vi "ExampleControl.vi"() -> ()   [LabVIEW 2017, in "Spectral Products CM110.lvlib"]
uses:
  Spectral Products CM110.lvlib
  Public/Controls/CaseSelector.ctl
panel:
  in  "Direction":bool caption="Clockwise"
  out "Rotation Speed":u16
  in  "Desired Rotation Speed":u16=1 min=1 step=1
  in  "Zero":bool
  in  "Desired Step Size":u8=1
  in  "Step":bool
  out "Step size":u8
  out "Changing grating":bool
  in  "Switch grating":bool
  out "Number of gratings":u8
  out "Groove Density":u16
  out "Blaze Wavelength":u16
  out "Current grating #":u8
  in  "Units":u8(ring)=1 items=["nm"=1, "A"=2]
  in  "Move Absolute":bool
  in  "Wavelength":u16
  out "Command not accepted":bool
  out "Error Out":errorcluster
  in  "QUIT":bool
  out "Position":cluster{"Numeric":dbl, "Units":string}
  out "Initialized":bool
  in  "VISA resource name":refnum<visa-resource-name>="COM7"
  # "CCW"
  # "CW"
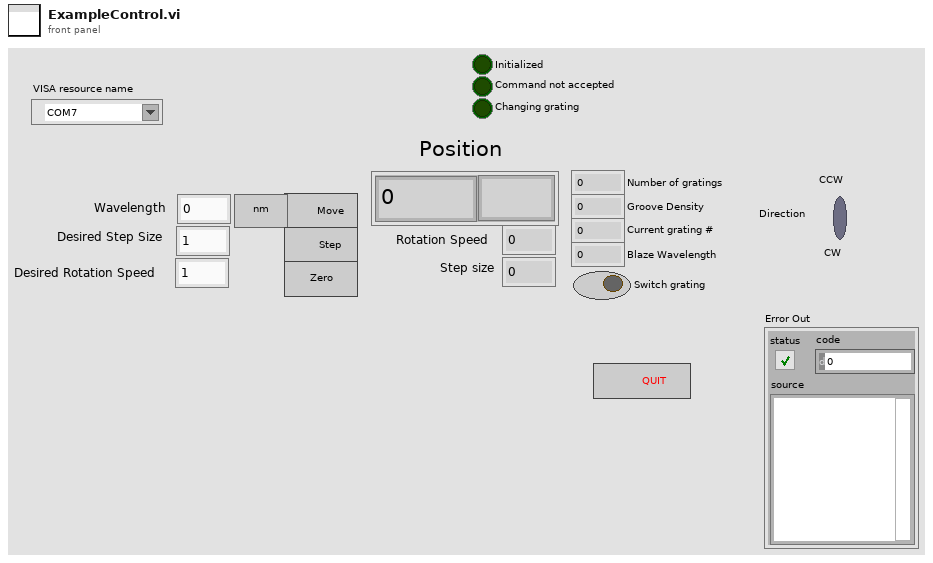
[diagram p1: front panel]
types:
  T1 = typedef "Spectral Products CM110.lvlib/CaseSelector.ctl" = enum16{"Initialize", "Get Status", "Idle", "Close", "GoTo", "Change Units", "Read Grating Info", "Change Grating", "Change Step Size", "Move One Step", "Reset", "Change Rotation Speed", "Change Rotation Direction"}
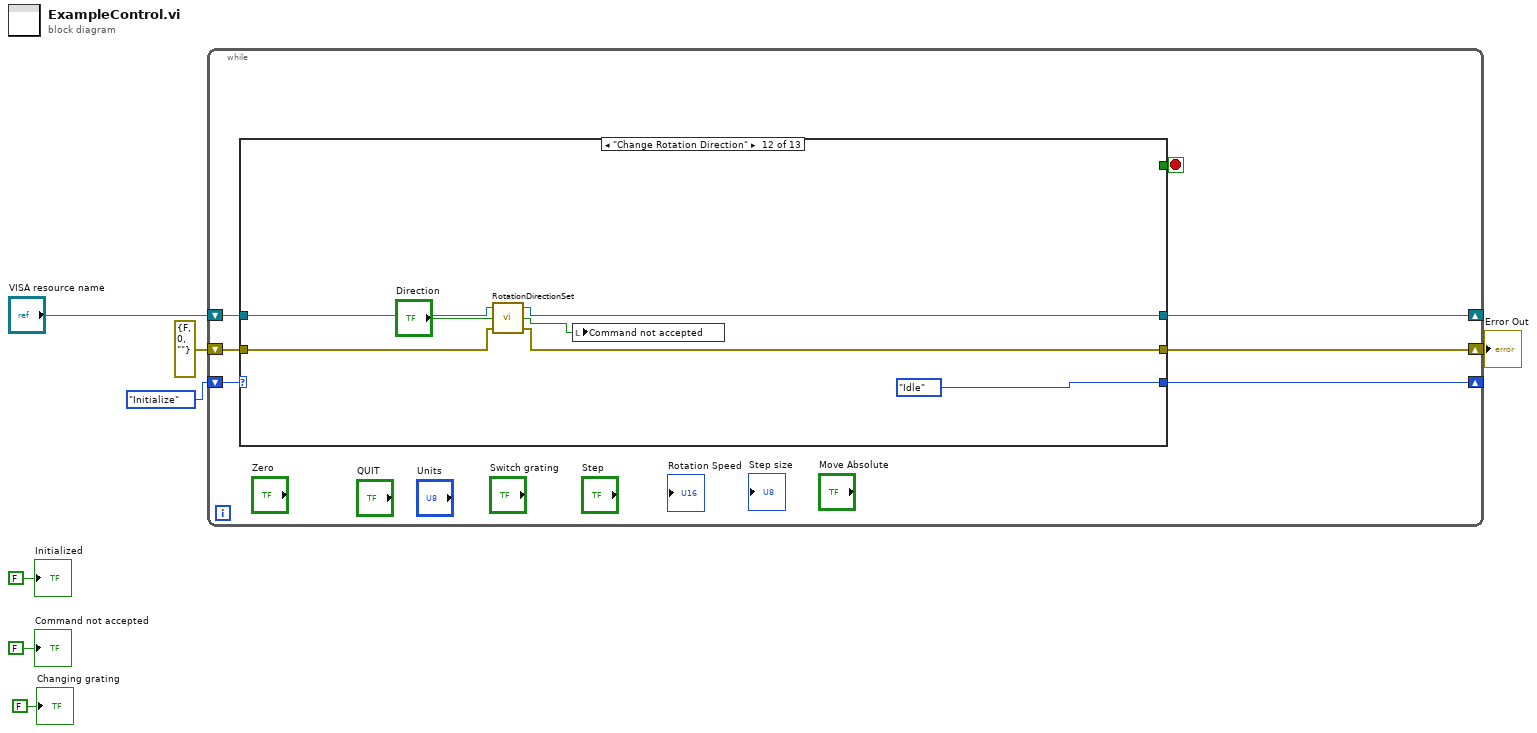
[diagram p0: block diagram]
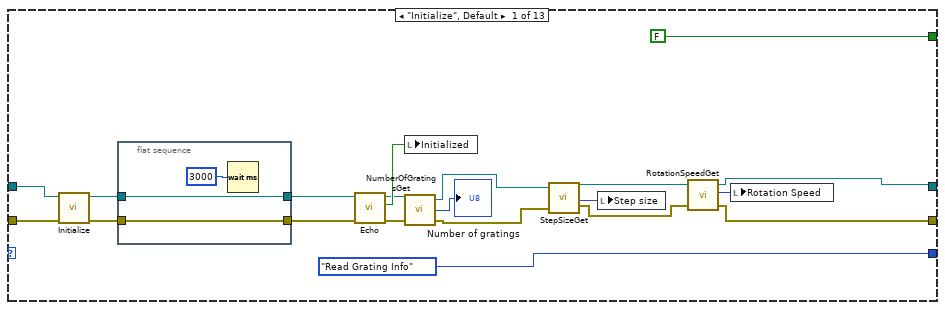
[diagram p2: hidden frame]
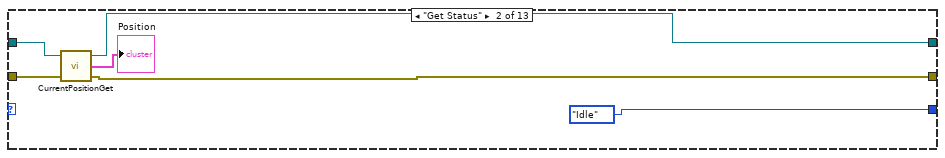
[diagram p3: hidden frame]
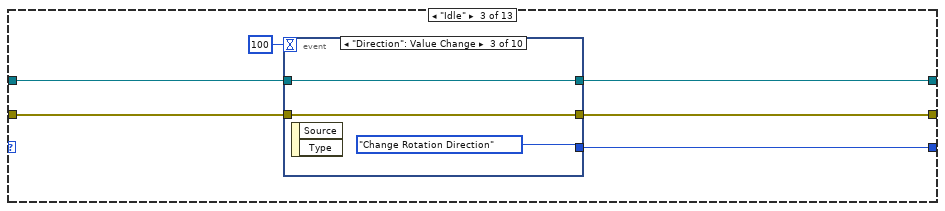
[diagram p4: hidden frame]
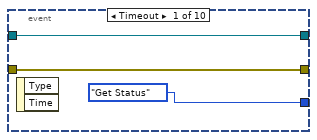
[diagram p5: hidden frame]
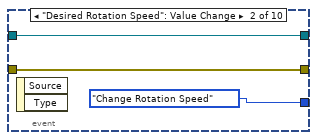
[diagram p6: hidden frame]
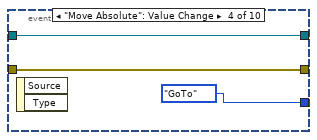
[diagram p7: hidden frame]
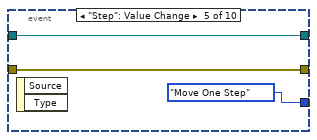
[diagram p8: hidden frame]
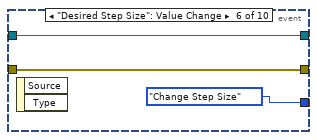
[diagram p9: hidden frame]
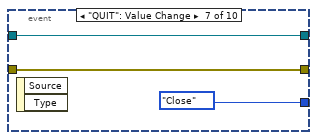
[diagram p10: hidden frame]
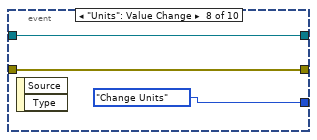
[diagram p11: hidden frame]
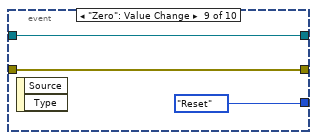
[diagram p12: hidden frame]
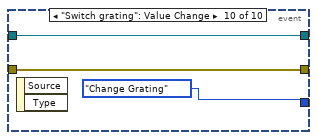
[diagram p13: hidden frame]
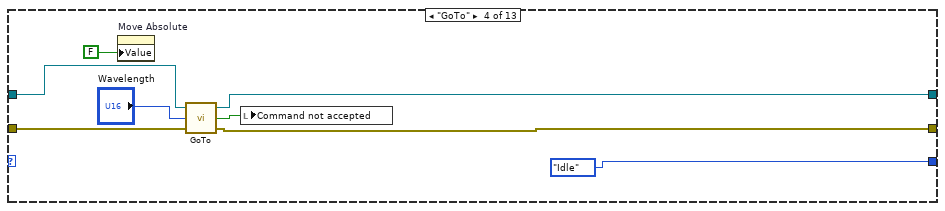
[diagram p14: hidden frame]
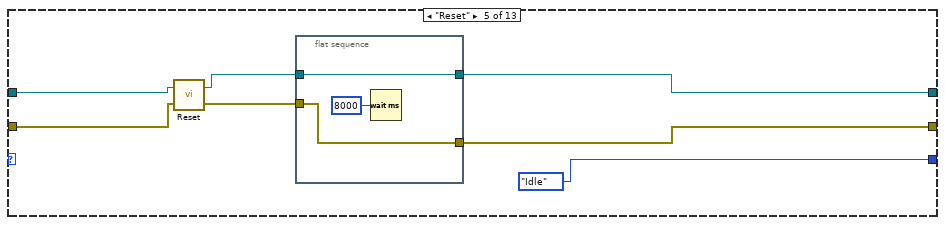
[diagram p15: hidden frame]
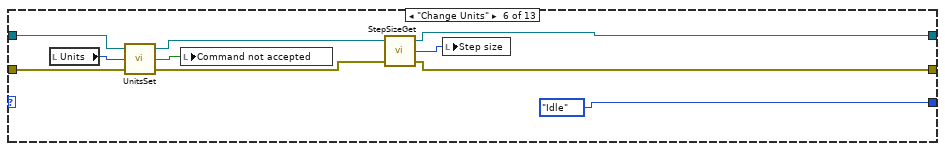
[diagram p16: hidden frame]
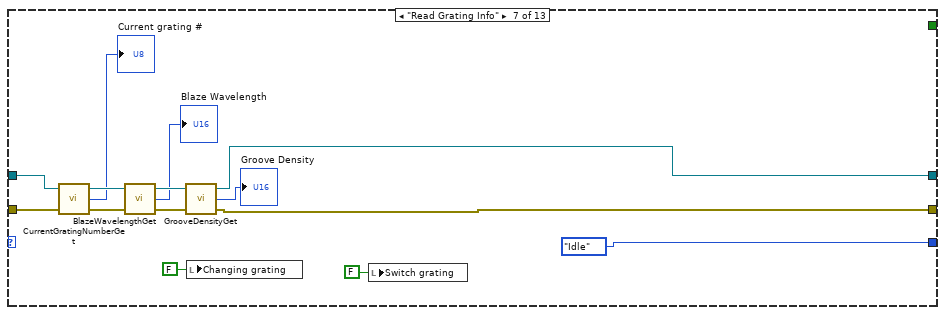
[diagram p17: hidden frame]
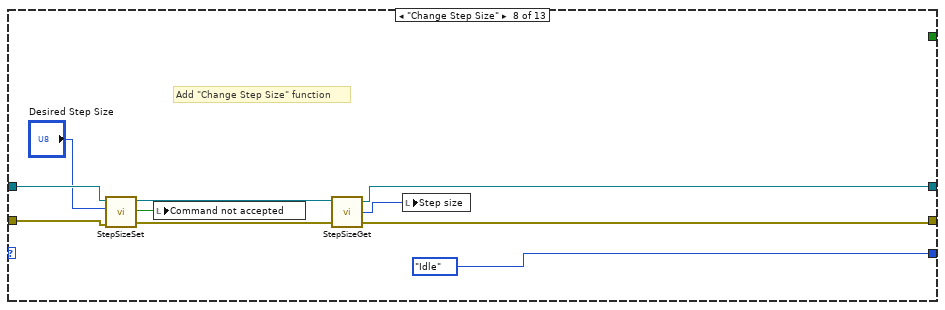
[diagram p18: hidden frame]
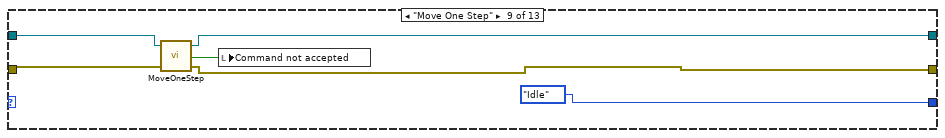
[diagram p19: hidden frame]
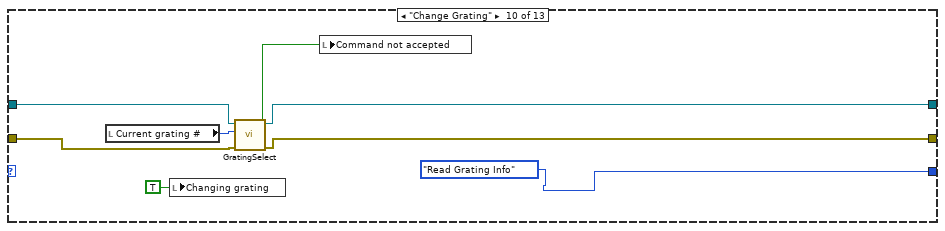
[diagram p20: hidden frame]
diagram:
  n1 = while {
    shift-right: [w11] -> _
    shift-left: "VISA resource name" -> [w14]
    shift-right: [w10] -> w3
    shift-left: errorcluster {"status"=FALSE, "code"=0, "source"=""} ("error in (no error)") -> [w13]
    shift-right: [w8] -> _
    shift-left: CaseSelector."Initialize" -> [w12]
    stop <- w9 stop-if-true
    n2 = case shown="\"Change Rotation Direction\"" w12 {
      tunnel: w14 -> [w34 w43 w46 w87 w94 w106 w121 w127 w136 w144 w155 w161 w166]
      tunnel: w13 -> [w33 w42 w44 w86 w93 w105 w120 w126 w135 w143 w153 w160 w168]
      tunnel: [w16 w40 w47 w82 w92 w99 w112 w131 w133 w141 w148 w158 w166] -> w11
      tunnel: [w15 w39 w45 w81 w90 w98 w111 w130 w132 w140 w147 w157 w165] -> w10
      tunnel: [FALSE ("Initialized") _ _ _ _ _ _ _ _ _ _ _ TRUE ("Initialized")] -> w9
      tunnel: [CaseSelector."Read Grating Info" CaseSelector."Idle" w48 CaseSelector."Idle" CaseSelector."Idle" CaseSelector."Idle" CaseSelector."Idle" CaseSelector."Idle" CaseSelector."Idle" CaseSelector."Read Grating Info" CaseSelector."Idle" CaseSelector."Idle" CaseSelector."Idle"] -> w8
      frame "Initialize", Default {
        n3 = call "Initialize.vi"("error in (no error)"=w33, "VISA resource name"=w34) -> ("error out"=w27:errorcluster, "VISA resource name out"=w28:refnum<visa-resource-name>)  [unwired: 8 in]
        n4 = flat-sequence {
          tunnel: w28 -> [w37]
          tunnel: [w37] -> w30
          tunnel: w27 -> [w36]
          tunnel: [w36] -> w29
          frame #0 {
            n5 = Wait (ms)(milliseconds to wait=u32 3000) -> ()  [unwired: 1 out]
          }
        }
        n6 = call "Echo.vi"("error in (no error)"=w29, "VISA resource name"=w30) -> ("error out"=w25:errorcluster, "ECHO"=w32:bool, "VISA resource name out"=w26:refnum<visa-resource-name>)  [unwired: 7 in]
        n7 = local write "Initialized"(w32) -> ()
        n8 = call "NumberOfGratingsGet.vi"("error in (no error)"=w25, "VISA resource name"=w26) -> ("error out"=w22:errorcluster, "Number of gratings"=→"Number of gratings":u8, "VISA resource name out"=w23:refnum<visa-resource-name>)  [unwired: 1 in]
        n9 = call "StepSizeGet.vi"("error in (no error)"=w22, "VISA resource name"=w23) -> ("error out"=w18:errorcluster, "Step size"=w20:u8, "VISA resource name out"=w19:refnum<visa-resource-name>)  [unwired: 1 in]
        n10 = local write "Step size"(w20) -> ()
        n11 = call "RotationSpeedGet.vi"("error in (no error)"=w18, "VISA resource name"=w19) -> ("error out"=w15:errorcluster, "Rotation Speed"=w17:u16, "VISA resource name out"=w16:refnum<visa-resource-name>)  [unwired: 1 in]
        n12 = local write "Rotation Speed"(w17) -> ()
      }
      frame "Get Status" {
        n13 = call "CurrentPositionGet.vi"("error in (no error)"=w42, "VISA resource name"=w43) -> ("error out"=w39:errorcluster, "Position"=→"Position":cluster{"Numeric":dbl, "Units":string}, "VISA resource name out"=w40:refnum<visa-resource-name>)  [unwired: 1 in]
      }
      frame "Idle" {
        n14 = event shown="[2] \"Direction\": Value Change" {
          selector: _ -> [_ _ _ _ _ _ _ _ _ _]
          dyn-events: _ -> [_ _ _ _ _ _ _ _ _ _]
          timeout: 100 -> [_ _ _ _ _ _ _ _ _ _]
          tunnel: [CaseSelector."Get Status" CaseSelector."Change Rotation Speed" CaseSelector."Change Rotation Direction" CaseSelector."GoTo" CaseSelector."Move One Step" CaseSelector."Change Step Size" CaseSelector."Close" CaseSelector."Change Units" CaseSelector."Reset" CaseSelector."Change Grating"] -> w48
          tunnel: [w52 w55 w56 w61 w62 w66 w70 w73 w76 w79] -> w47
          tunnel: w46 -> [w52 w55 w56 w61 w62 w66 w70 w73 w76 w79]
          tunnel: [w51 w54 w57 w60 w63 w65 w69 w72 w75 w78] -> w45
          tunnel: w44 -> [w51 w54 w57 w60 w63 w65 w69 w72 w75 w78]
          event Timeout {
            n15 = event-data() -> ()  [unwired: 1 in, 2 out]
          }
          event "Desired Rotation Speed": Value Change {
            n16 = event-data() -> ()  [unwired: 1 in, 2 out]
          }
          event "Direction": Value Change {
            n17 = event-data() -> ()  [unwired: 1 in, 2 out]
          }
          event "Move Absolute": Value Change {
            n18 = event-data() -> ()  [unwired: 1 in, 2 out]
          }
          event "Step": Value Change {
            n19 = event-data() -> ()  [unwired: 1 in, 2 out]
          }
          event "Desired Step Size": Value Change {
            n20 = event-data() -> ()  [unwired: 1 in, 2 out]
          }
          event "QUIT": Value Change {
            n21 = event-data() -> ()  [unwired: 1 in, 2 out]
          }
          event "Units": Value Change {
            n22 = event-data() -> ()  [unwired: 1 in, 2 out]
          }
          event "Zero": Value Change {
            n23 = event-data() -> ()  [unwired: 1 in, 2 out]
          }
          event "Switch grating": Value Change {
            n24 = event-data() -> ()  [unwired: 1 in, 2 out]
          }
        }
      }
      frame "GoTo" {
        n25 = property on="Move Absolute" class="Bool (strict)"("Value"=FALSE ("Move Absolute")) -> ()  [unwired: 2 in, 2 out]
        n26 = call "GoTo.vi"("error in (no error)"=w86, "Wavelength"="Wavelength", "VISA resource name"=w87) -> ("error out"=w81:errorcluster, "Command not accepted"=w84:bool, "VISA resource name out"=w82:refnum<visa-resource-name>)
        n27 = local write "Command not accepted"(w84) -> ()
      }
      frame "Reset" {
        n28 = call "Reset.vi"("error in (no error)"=w93, "VISA resource name"=w94) -> ("error out"=w89:errorcluster, "VISA resource name out"=w91:refnum<visa-resource-name>)
        n29 = flat-sequence {
          tunnel: [w96] -> w92
          tunnel: w91 -> [w96]
          tunnel: [w95] -> w90
          tunnel: w89 -> [w95]
          frame #0 {
            n30 = Wait (ms)(milliseconds to wait=u32 8000) -> ()  [unwired: 1 out]
          }
        }
      }
      frame "Change Units" {
        n31 = local read "Units"() -> (w107:u8)
        n32 = call "UnitsSet.vi"("error in (no error)"=w105, "Units"=w107, "VISA resource name"=w106) -> ("error out"=w101:errorcluster, "Command not accepted"=w104:bool, "VISA resource name out"=w102:refnum<visa-resource-name>)
        n33 = local write "Command not accepted"(w104) -> ()
        n34 = call "StepSizeGet.vi"("error in (no error)"=w101, "VISA resource name"=w102) -> ("error out"=w98:errorcluster, "Step size"=w100:u8, "VISA resource name out"=w99:refnum<visa-resource-name>)  [unwired: 1 in]
        n35 = local write "Step size"(w100) -> ()
      }
      frame "Read Grating Info" {
        n36 = call "CurrentGratingNumberGet.vi"("error in (no error)"=w120, "VISA resource name"=w121) -> ("error out"=w118:errorcluster, "Current grating #"=→"Current grating #":u8, "VISA resource name out"=w119:refnum<visa-resource-name>)  [unwired: 1 in]
        n37 = call "BlazeWavelengthGet.vi"("error in (no error)"=w118, "VISA resource name"=w119) -> ("error out"=w116:errorcluster, "Blaze Wavelength"=→"Blaze Wavelength":u16, "VISA resource name out"=w117:refnum<visa-resource-name>)  [unwired: 1 in]
        n38 = call "GrooveDensityGet.vi"("error in (no error)"=w116, "VISA resource name"=w117) -> ("error out"=w111:errorcluster, "Groove Density"=→"Groove Density":u16, "VISA resource name out"=w112:refnum<visa-resource-name>)  [unwired: 1 in]
        n39 = local write "Changing grating"(FALSE ("Changing grating")) -> ()
        n40 = local write "Switch grating"(FALSE ("Switch grating")) -> ()
      }
      frame "Change Step Size" {
        # "Add \"Change Step Size\" function"
        n41 = call "StepSizeSet.vi"("error in (no error)"=w126, "Desired Step Size"="Desired Step Size", "VISA resource name"=w127) -> ("error out"=w123:errorcluster, "Command not accepted"=w122:bool, "VISA resource name out"=w124:refnum<visa-resource-name>)  [unwired: 6 in]
        n42 = local write "Command not accepted"(w122) -> ()
        n43 = call "StepSizeGet.vi"("error in (no error)"=w123, "VISA resource name"=w124) -> ("error out"=w130:errorcluster, "Step size"=w129:u8, "VISA resource name out"=w131:refnum<visa-resource-name>)  [unwired: 1 in]
        n44 = local write "Step size"(w129) -> ()
      }
      frame "Move One Step" {
        n45 = call "MoveOneStep.vi"("error in (no error)"=w135, "VISA resource name"=w136) -> ("error out"=w132:errorcluster, "Command not accepted"=w134:bool, "VISA resource name out"=w133:refnum<visa-resource-name>)  [unwired: 1 in]
        n46 = local write "Command not accepted"(w134) -> ()
      }
      frame "Change Grating" {
        n47 = local read "Current grating #"() -> (w145:u8)
        n48 = local write "Changing grating"(TRUE ("Changing grating")) -> ()
        n49 = call "GratingSelect.vi"("error in (no error)"=w143, "Current Grating"=w145, "VISA resource name"=w144) -> ("error out"=w140:errorcluster, "Command not accepted"=w142:bool, "VISA resource name out"=w141:refnum<visa-resource-name>)  [unwired: 6 in]
        n50 = local write "Command not accepted"(w142) -> ()
      }
      frame "Change Rotation Speed" {
        n51 = call "RotationSpeedSet.vi"("error in (no error)"=w153, "Rotation Speed"="Desired Rotation Speed", "VISA resource name"=w155) -> ("error out"=w149:errorcluster, "Command not accepted"=w152:bool, "VISA resource name out"=w150:refnum<visa-resource-name>)
        n52 = local write "Command not accepted"(w152) -> ()
        n53 = call "RotationSpeedGet.vi"("error in (no error)"=w149, "VISA resource name"=w150) -> ("error out"=w147:errorcluster, "Rotation Speed"=w146:u16, "VISA resource name out"=w148:refnum<visa-resource-name>)  [unwired: 1 in]
        n54 = local write "Rotation Speed"(w146) -> ()
      }
      frame "Change Rotation Direction" {
        n55 = call "RotationDirectionSet.vi"("error in (no error)"=w160, "Counterclockwise"="Direction", "VISA resource name"=w161) -> ("error out"=w157:errorcluster, "Command not accepted"=w156:bool, "VISA resource name out"=w158:refnum<visa-resource-name>)
        n56 = local write "Command not accepted"(w156) -> ()
      }
      frame "Close" {
        n57 = call "Close.vi"("error in (no error)"=w168, "VISA resource name"=w166) -> ("error out"=w165:errorcluster)  [unwired: 9 in]
        n58 = local write "QUIT"(FALSE ("QUIT")) -> ()
      }
    }
  }
  "Error Out" <- w3
  "Initialized" <- FALSE ("Initialized")
  "Command not accepted" <- FALSE ("Command not accepted")
  "Changing grating" <- FALSE ("Changing grating")
